vi "Configure Timing.vi"(8 "error in (no error)":errorcluster, 11 "Thermometer DAQmx Config in":refnum<class "Thermometer DAQmx Config.lvclass">) -> (0 "error out":errorcluster, 3 "Thermometer DAQmx Config out":refnum<class "Thermometer DAQmx Config.lvclass">)   [LabVIEW 2023, in "Thermometer.lvlib" / "Thermometer DAQmx.lvlib" / "Thermometer DAQmx Config.lvclass"]
uses:
  Thermometer DAQmx Config.lvclass
  Configuration Base/Configuration Base.lvclass/Configuration Base.ctl
  Thermometer DAQmx Config.lvclass/Thermometer DAQmx Config.ctl
  6a24a77e-4e51-482f-9e0f-1e54414336e5.vi
  bb6916d1-18ad-4f5c-a7cb-916ce281d5be.vi
  14682934-d4ee-47d1-b4c2-e729f8facd9e.vi
  <vilib>/JDP Science/JSONtext/Next JSON Value.vi
  <vilib>/JDP Science/JSONtext/String Subset.vi
  <vilib>/JDP Science/JSONtext/Parsing/Advance past next JSON Value (inlined COPY).vi
  <vilib>/JDP Science/JSONtext/Parsing/Advance past whitespace.vi
  <vilib>/JDP Science/JSONtext/Parsing/Advance past String.vi
  <vilib>/JDP Science/JSONtext/Parsing/Advance past Number.vi
  <vilib>/JDP Science/JSONtext/Parsing/Advance past Line Ending.vi
  <vilib>/JDP Science/JSONtext/Parsing/Parse Full Path or Item Name.vi
  <vilib>/JDP Science/JSONtext/Parsing/Advance past Array.vi
  <vilib>/JDP Science/JSONtext/Parsing/Advance past Object.vi
  <vilib>/JDP Science/JSONtext/support/Error Cluster From Code.vi
  <vilib>/JDP Science/JSONtext/Offset/Find Item Locations by Path.vi
  <vilib>/JDP Science/JSONtext/JSON text to Variant.vi
  <vilib>/Utility/error.llb/Error Cluster From Error Code.vi
  <vilib>/DAQmx/configure/timing.llb/DAQmx Timing (Sample Clock).vi
  <vilib>/JDP Science/JSONtext/LVClass Serializer/JSONtext LVClass Serializer.lvclass
  <vilib>/ErrorRing/Error Ring.xnode
  Configuration Base/Configuration Base.lvclass
  <resource>/objmgr/daqmx.rc
  <vilib>/JDP Science/JSONtext/JSONtext.lvlib
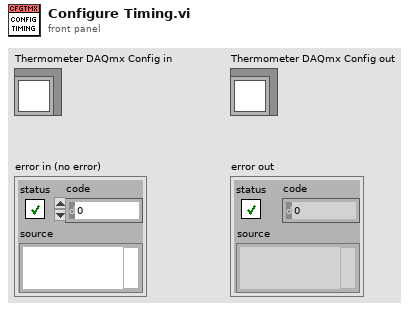
[diagram p1: front panel]
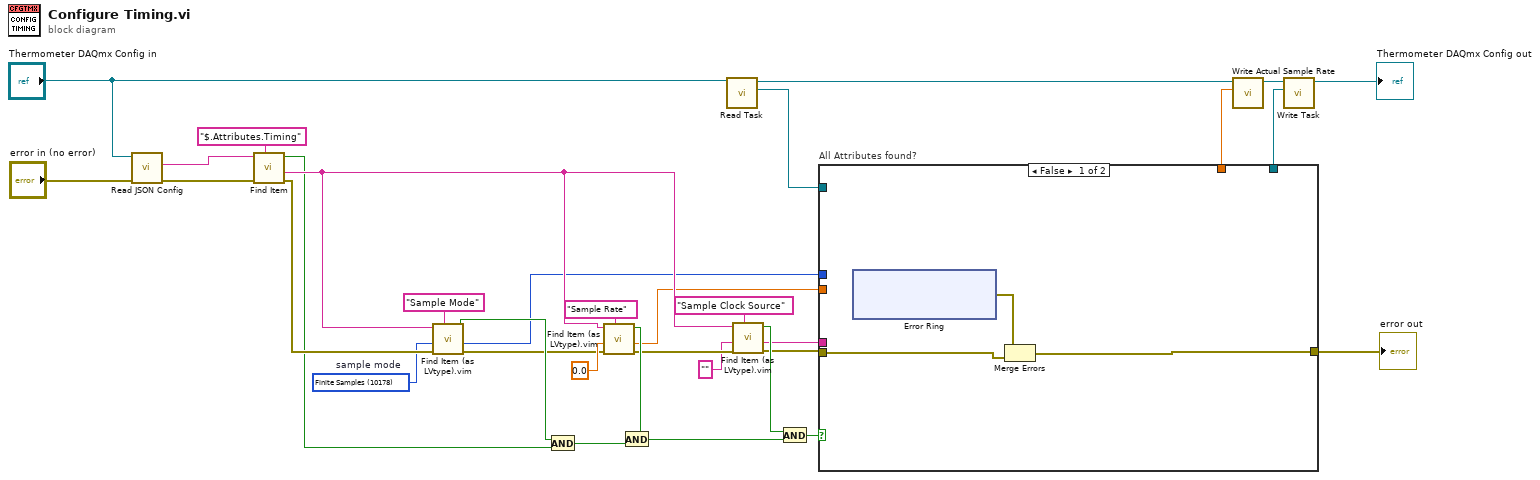
[diagram p0: block diagram]
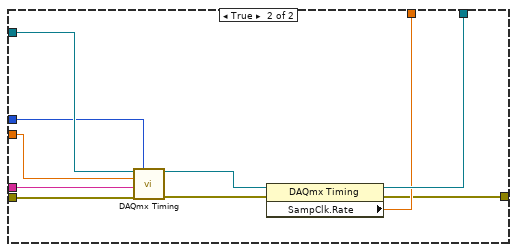
[diagram p2: hidden frame]
diagram:
  w1 = 10178 items=["Finite Samples"=10178, "Continuous Samples"=10123, "Hardware Timed Single Point"=12522]  # sample mode
  n1 = call "Read JSON Config.vi"("error in"="error in (no error)", "object in"="Thermometer DAQmx Config in") -> ("error out"=w33:errorcluster, "<JSON>Config"=w32:string)  [unwired: 7 in, 1 out]
  n2 = call <vilib>:"Find Item.vi"("$Path or Item Name"="$.Attributes.Timing", "error in (no error)"=w33, "JSON"=w32) -> ("error out"=w31:errorcluster, "<JSON>"=w29:string, "Found"=w4:bool)  [unwired: 5 in, 1 out]
  n3 = call "Find Item (as LVtype).vim"("$Path or Item Name"="Sample Mode", "error in (no error)"=w31, "Data Type and Default Value"=w1, "JSON"=w29) -> ("error out"=w3:errorcluster, "Data"=w2:i32, "Found"=w20:bool)  [unwired: 4 in, 1 out]
  n4 = And(x=w20, y=w4) -> (x .and. y?=w18:bool)
  n5 = call "Find Item (as LVtype).vim"("$Path or Item Name"="Sample Rate", "error in (no error)"=w3, "Data Type and Default Value"=0.0, "JSON"=w29) -> ("error out"=w17:errorcluster, "Data"=w10:dbl, "Found"=w19:bool)  [unwired: 4 in, 1 out]
  n6 = And(x=w19, y=w18) -> (x .and. y?=w9:bool)
  n7 = call "Read Task.vi"("Thermometer DAQmx Config in"="Thermometer DAQmx Config in") -> ("Task"=w27:refnum<k21>, "Thermometer DAQmx Config out"=w28:refnum<class "Thermometer DAQmx Config.lvclass">)  [unwired: 8 in, 1 out]
  n8 = call "Find Item (as LVtype).vim"("$Path or Item Name"="Sample Clock Source", "error in (no error)"=w17, "Data Type and Default Value"="" ("Auto Zero Mode"), "JSON"=w29) -> ("error out"=w11:errorcluster, "Data"=w12:string, "Found"=w13:bool)  [unwired: 4 in, 1 out]
  n9 = And(x=w13, y=w9) -> (x .and. y?=w14:bool)
  n10 = case "All Attributes found?" shown="False" w14 {
    tunnel: w11 -> [w34 w51]
    tunnel: [w35 w44] -> w24
    tunnel: w27 -> [_ w49]
    tunnel: w12 -> [_ w43]
    tunnel: w10 -> [_ w50]
    tunnel: w2 -> [_ w42]
    tunnel: [_ w46] -> w7
    tunnel: [_ w45] -> w5
    frame False {
      n11 = xnode "Error Ring"() -> ("error out"=w36:errorcluster)
      n12 = Merge Errors(w36, w34) -> (w35:errorcluster)
    }
    frame True {
      n13 = call-poly <vilib>:"DAQmx Timing.vi"("task/channels in"=w49, "sample mode"=w42, "rate"=w50, "source"=w43, "error in"=w51) -> ("task out"=w47:refnum<k21>, "error out"=w48:errorcluster)  [unwired: 9 in]
      n14 = property class="DAQmx Timing"(reference=w47, error in=w48) -> (reference out=w46:refnum<k21>, error out=w44:errorcluster, "SampClk.Rate"=w45:dbl)
    }
  }
  "error out" <- w24
  n15 = call "Write Actual Sample Rate.vi"("Actual Sample Rate"=w5, "Thermometer DAQmx Config in"=w28) -> ("Thermometer DAQmx Config out"=w6:refnum<class "Thermometer DAQmx Config.lvclass">)  [unwired: 8 in, 1 out]
  n16 = call "Write Task.vi"("Task"=w7, "Thermometer DAQmx Config in"=w6) -> ("Thermometer DAQmx Config out"=→"Thermometer DAQmx Config out":refnum<class "Thermometer DAQmx Config.lvclass">)  [unwired: 8 in, 1 out]
